vi "WPI_DashboardGet All Users Directory.vi"() -> (0 "All User Path":path)   [LabVIEW 2025]
uses:
  <vilib>/Utility/sysdir.llb/System Directory Type.ctl
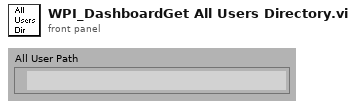
[diagram p1: front panel]
types:
  T1 = typedef "System Directory Type.ctl" = i32
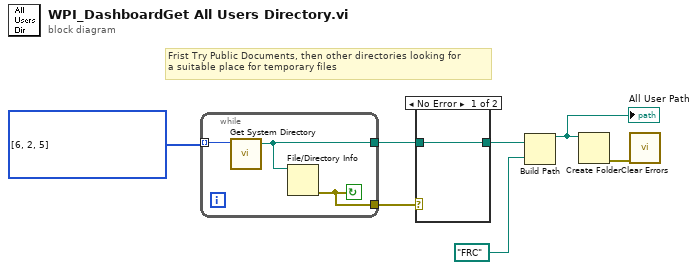
[diagram p0: block diagram]
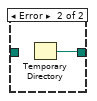
[diagram p2: hidden frame]
diagram:
  w7 = T1[] [6, 2, 5] items=["User Home"=0, "User Desktop"=1, "User Documents"=2, "User Application Data"=3, "User Preferences"=4, "User Temporary"=5, "Public Documents"=6, "Public Application Data"=7, "Public Preferences"=8, "Public Cache"=13, "System Core Libraries"=9, "System Installed Libraries"=10, "Application Files"=11, "Boot Volume Root"=12]
  # "Frist Try Public Documents, then other directories looking for\na suitable place for temporary files"
  n1 = while {
    tunnel: [w9] -> w5
    tunnel: w7 -> [w10] mode=indexing
    tunnel: [w8] -> w6
    stop <- w8 continue-if-true
    n2 = call <vilib>:"Get System Directory.vi"("system directory type"=w10) -> ("system directory"=w9:path)  [unwired: 10 in]
    n3 = File/Directory Info(path=w9) -> (error out=w8:errorcluster)  [unwired: 1 in, 6 out]
  }
  n4 = case shown="No Error" w6 {
    tunnel: w5 -> [w11 _]
    tunnel: [w11 w12] -> w4
    frame No Error {
    }
    frame Error {
      n5 = Temporary Directory() -> (w12:path)
    }
  }
  n6 = Build Path(base path=w4, name or relative path=path "FRC") -> (appended path=w2:path)
  "All User Path" <- w2
  n7 = Create Folder(path (use dialog)=w2) -> (error out=w1:errorcluster)  [unwired: 2 in, 2 out]
  n8 = call <vilib>:"Clear Errors.vi"("error in (no error)"=w1) -> ()  [unwired: 5 in, 2 out]
